vi "search-pannel-from-id.vi"(10 "pannel-id":dbl, 11 "sce-pannel-list":T2(array[cluster])) -> (3 "sce-pannel":T1)   [LabVIEW 2019]
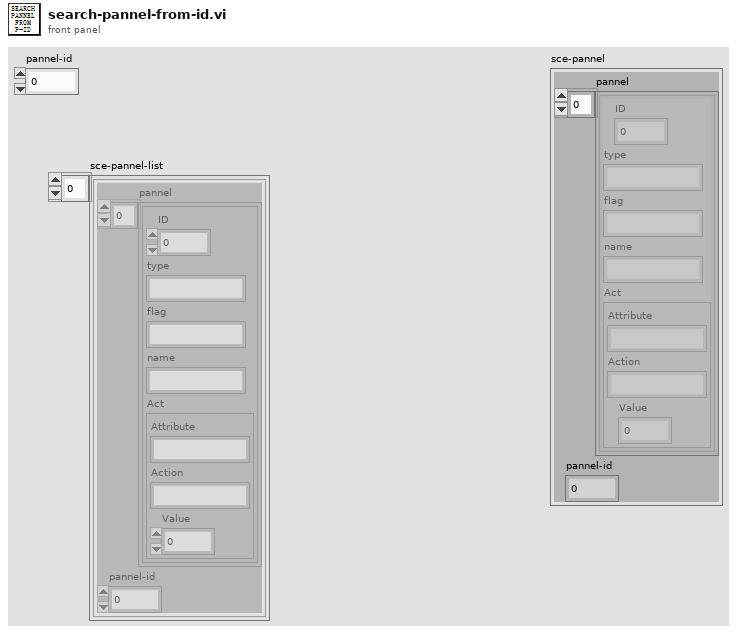
[diagram p1: front panel]
types:
  T1 = cluster{"pannel":cluster{"ID":u8, "type":string, "flag":string, "name":string, "Act":cluster{"Attribute":string, "Action":string, "Value":dbl}}[], "pannel-id":dbl}
  T2 = cluster{"pannel":cluster{"ID":u8, "type":string, "flag":string, "name":string, "Act":cluster{"Attribute":string, "Action":string, "Value":dbl}}[], "pannel-id":dbl}[]
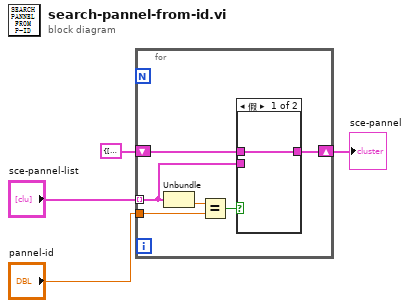
[diagram p0: block diagram]
diagram:
  n1 = for {
    tunnel: "sce-pannel-list" -> [w6] mode=indexing
    shift-right: [w7] -> w1
    shift-left: T1 {"pannel"=[], "pannel-id"=-1.0} ("sce-pannel") -> [w5]
    tunnel: "pannel-id" -> [w9]
    n2 = Unbundle(w6) -> ("pannel-id"=w10:dbl)  [unwired: 1 out]
    n3 = Equal?(x=w10, y=w9) -> (x = y?=w8:bool)
    n4 = case shown="假" w8 {
      tunnel: [w11 w12] -> w7
      tunnel: w6 -> [_ w12]
      tunnel: w5 -> [w11 _]
      frame False {
      }
      frame True {
      }
    }
  }
  "sce-pannel" <- w1
